vi "zad4.vi"() -> ()   [LabVIEW 2018]
panel:
  out "String":string
  out "Waveform Chart":i32(graph)
  out "concatenated string":string
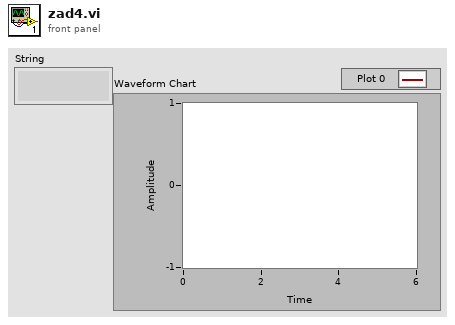
[diagram p1: front panel]
types:
  T1 = enum16{"Standard", "Buffered", "CRLF", "Immediate"}
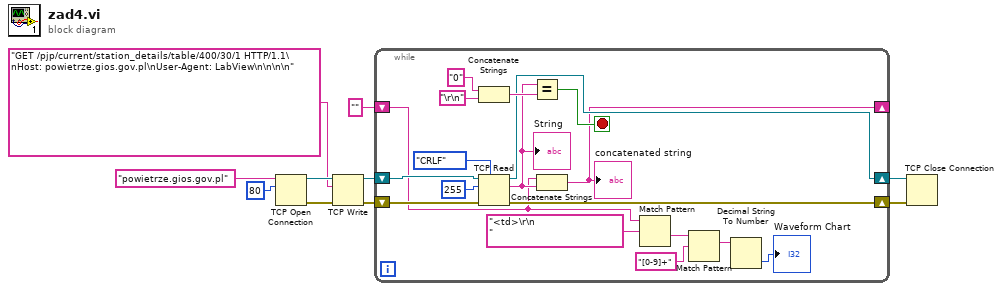
[diagram p0: block diagram]
diagram:
  n1 = TCP Open Connection(address="powietrze.gios.gov.pl", remote port or service name=u16 80) -> (connection ID=w9:refnum<k5>, error out=w10:errorcluster)  [unwired: 3 in]
  n2 = TCP Write(connection ID=w9, data in="GET /pjp/current/station_details/table/400/30/1 HTTP/1.1\nHost: powietrze.gios.gov.pl\nUser-Agent: LabView\n\n\n\n", error in (no error)=w10) -> (connection ID out=w5:refnum<k5>, error out=w4:errorcluster)  [unwired: 1 in, 1 out]
  n3 = while {
    shift-right: [w17] -> _
    shift-left: "" -> [w11]
    shift-right: [w21] -> w3
    shift-left: w4 -> [w27]
    shift-right: [w19] -> w2
    shift-left: w5 -> [w28]
    stop <- w24 stop-if-true
    n4 = Concatenate Strings("0" ("string"), "\r\n") -> (w23:string)
    n5 = TCP Read(connection ID=w28, bytes to read=255, error in (no error)=w27, 7:T1."CRLF" ("mode (standard)")) -> (connection ID out=w19:refnum<k5>, data out=w18:string, error out=w21:errorcluster)  [unwired: 1 in]
    "String" <- w18
    n6 = Equal?(x=w18, y=w23) -> (x = y?=w24:bool)
    n7 = Concatenate Strings(w11, w18) -> (w17:string)
    "concatenated string" <- w17
    n8 = Match Pattern(string=w11, regular expression="<td>\r\n                                           ") -> (after substring=w15:string)  [unwired: 1 in, 3 out]
    n9 = Match Pattern(string=w15, regular expression="[0-9]+") -> (match substring=w13:string)  [unwired: 1 in, 3 out]
    n10 = Decimal String To Number(string=w13) -> (number=→"Waveform Chart":i32)  [unwired: 2 in, 1 out]
  }
  n11 = TCP Close Connection(connection ID=w2, error in (no error)=w3) -> ()  [unwired: 1 in, 2 out]
